vi "Complex Array - Does Not Contain.vi"() -> ()   [LabVIEW 2017, in "Assertions.Tests.lvlib" / "Assert Collection Not Contains.lvlib"]
uses:
  Assert Collection Not Contains.lvlib
  src/Transparent Assertions/Constraints/Collection Contains/Collection Contains.lvclass
  C:/Users/pasca/Projects/Home/TransparentAssertions/src/Transparent Assertions/Constraints/Constraint/Constraint.lvclass
  src/Transparent Assertions/Constraints/Collection Contains/Create.vi
  src/Transparent Assertions/Constraints/LogicalNot/LogicalNot.lvclass
  src/Transparent Assertions/Constraints/UnaryOperator/UnaryOperator.lvclass
  src/Transparent Assertions/Assertions/Assertions.lvlib
panel:
  out "error out":errorcluster
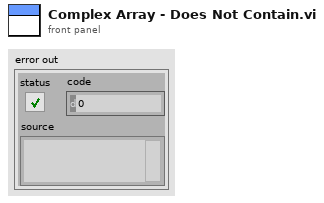
[diagram p1: front panel]
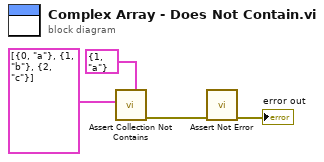
[diagram p0: block diagram]
diagram:
  n1 = call "Assert Collection Not Contains.vi"("Expected"=cluster{i32, string} {1, "a"}, "Collection"=cluster{i32, string}[] [{0, "a"}, {1, "b"}, {2, "c"}]) -> ("error out"=w1:errorcluster)  [unwired: 9 in]
  n2 = call "Assert Not Error.vi"("error in (no error)"=w1) -> ("error out"=→"error out":errorcluster)  [unwired: 10 in]
